vi "MasterAquisitionFile_IOS_Optogenetics_test_no_DigitalOutput.vi"() -> ()   [LabVIEW 2018]
uses:
  <vilib>/vision/driver/IMAQdx.llb/IMAQdx Acquisition Mode.ctl
  <vilib>/vision/driver/IMAQdx.llb/IMAQdx Camera Control Mode.ctl
  <vilib>/userdefined/High Color/IMAQdx.ctl
  <vilib>/vision/driver/IMAQdx.llb/IMAQdx Buffer Number Mode.ctl
  <vilib>/DAQmx/write.llb/DAQmx Write (Analog 2D DBL NChan NSamp).vi
  <vilib>/DAQmx/write.llb/DAQmx Write (Digital Bool 1Line 1Point).vi
  <vilib>/DAQmx/read.llb/DAQmx Read (Analog 1D Wfm NChan NSamp).vi
  <vilib>/DAQmx/create/channels.llb/DAQmx Create Channel (DO-Digital Output).vi
  <vilib>/DAQmx/create/channels.llb/DAQmx Create Channel (AO-Voltage-Basic).vi
  <vilib>/DAQmx/create/channels.llb/DAQmx Create Channel (CO-Pulse Generation-Frequency).vi
  <vilib>/DAQmx/configure/timing.llb/DAQmx Timing (Implicit).vi
  <vilib>/DAQmx/create/channels.llb/DAQmx Create Channel (AI-Voltage-Basic).vi
  <vilib>/DAQmx/configure/timing.llb/DAQmx Timing (Sample Clock).vi
  <vilib>/DAQmx/configure/trigger.llb/DAQmx Start Trigger (Digital Edge).vi
  <vilib>/DAQmx/miscellaneous.llb/DAQmx Fill In Error Info.vi
  <vilib>/vision/driver/NI_Vision_Acquisition_Software.lvlib
  <resource>/objmgr/imaqdx.rc
  <resource>/objmgr/daqmx.rc
panel:
  in  "Solenoid\nPulse Train":bool=TRUE
  out "LED":bool
  out "Auditory":bool
  out "RPad":bool
  out "LPad":bool
  out "Finished":bool
  in  "LED":bool=TRUE
  in  "Sol Stim Parameters":cluster{"Fs":dbl, "Samples":dbl}
  in  "LED Stim Parameters":cluster{"Fs":dbl, "Samples":dbl}
  in  "Sol Duty Cycle (%)":dbl=10.0
  in  "Sol Freq":dbl=1.0
  in  "Sol Dur (s)":dbl=1.0
  in  "LED Duty Cycle (%)":dbl=10.0
  in  "LED Freq":dbl=10.0
  in  "LED Dur (s)":dbl=2.0
  out "Stimulus Order":digitalwaveform[](graph)=[{"t0"=timestamp(0 s since 1904-01-01), "dt"=5e-05, "Y"={"transitions"=[], "data"=array18000000x1[18000000 elements]}}, {"t0"=timestamp(0 s since 1904-01-01), "dt"=5e-05, "Y"={"transitions"=[], "data"=array18000000x1[18000000 elements]}}, {"t0"=timestamp(0 s since 1904-01-01), "dt"=5e-05, "Y"={"transitions"=[], "data"=array18000000x1[18000000 elements]}}, {"t0"=timestamp(0 s since 1904-01-01), "dt"=5e-05, "Y"={"transitions"=[], "data"=array18000000x1[18000000 elements]}}]
  out "Solenoid Stim":digitalwaveform(graph)={"t0"=timestamp(0 s since 1904-01-01), "dt"=5e-05, "Y"={"transitions"=[], "data"=array20000x1[20000 elements]}}
  in  "Trial Offset (s)":dbl=15.0
  in  "Interstim (s)":dbl=30.0
  in  "Right Pad":dbl=1.0
  in  "Left Pad":dbl=1.0
  in  "Auditory":dbl=1.0
  in  "LED":dbl
  out "Dev2 Samples":i32=526603
  out "Dev2 Analog":bool=TRUE
  in  "Dev2 Analog Channels":string[](array[string])=["LD_BackScatter", "LD_Flow", "Opto_LED", "RPadSol", "AudSol", "Hippocampus", "EMG", "Cortical_RH"]
  out "?":T1(plugin-control)
  out "?":T1(plugin-control)
  out "?":T1(plugin-control)
  out "?":T1(plugin-control)
  in  "stop":bool
  out "CBV Cam":bool=TRUE
  out "Pupil Cam":bool=TRUE
  out "Whisk Cam":bool=TRUE
  out "Web Cam":bool=TRUE
  out "Dev1 Analog":bool=TRUE
  out "Web Cam Fs":dbl(knob)=29.14753443801158 scale=0.0..200.0
  out "CBV Cam":dbl(knob)=30.019685039370078 scale=0.0..200.0
  out "Whisk Cam Fs":dbl(knob)=150.04985044865404 scale=0.0..200.0
  out "Last Whisk\nBuffer 2":u32=789
  out "Pupil Cam Fs":dbl(knob)=29.985007496251875 scale=0.0..200.0
  out "Dropped 2":u32(slide) caption="Pupil Cam" scale=0.0..99.0
  in  "Exposure Time (microsec)":string="10000"
  out "Dev1 Samples":i32=526592
  in  "Dev1 Analog Channels":string[](array[string])=["Cortical_LH", "Force_Sensor", "LPadSol", "RPadSol", "AudSol", "Hippocampus", "EMG", "Cortical_RH"]
  in  "Analog Acquisition":cluster{"Analog Fs":u16}={"Analog Fs"=20000} {"Analog Fs" format="%0.0f"}
  in  "Sampling Rates":T2={"CBV Cam Fs"=30, "Whisk Cam Fs"=150, "Web Cam Fs"=15, "Pupil Cam Fs"=30}
  out "Notes Size":i32=8
  out "Notes Reversed":string[](array[string])=["Experimenter", "Animal ID", "Hemisphere", "Solenoid PSI", "Isoflurane time", "Session ID", "Amplifier Gain", "LED power (mW)"]
  out "Notes Array":string[](array[string])=["LED power (mW)", "Amplifier Gain", "Session ID", "Isoflurane time", "Solenoid PSI", "Hemisphere", "Animal ID", "Experimenter"]
  in  "Notes:":T3={"Experimenter"="Kevin", "Animal ID"="T182", "Hemisphere"="Both", "Solenoid PSI"="10", "Isoflurane time"="1030", "Session ID"="Imaging Session Two", "Amplifier Gain"="10000", "LED power (mW)"="0"}
  in  "Target Path":path=path "D:/T182/Imaging Session 2 - 20 Apr. 2021" caption="Final Save Location"
  out "Dropped":u32(slide) caption="Whisk Cam" scale=0.0..999.0
  out "Filename":string="210420_10_44_31"
  out "CBV Camera":bool
  out "Time Elapsed (Min)":cluster{dbl, dbl}(slide)={15.0, 0.43888776} scale=0.0..15.0 scale format="%#_2g"
  in  "Time (min)":dbl(knob)=15.0 min=0.5 max=20.0 step=0.5 scale=0.0..20.0 scale format="%#_2g"
  in  "Temp Path":path=path "D:/LabVIEW Streamed Data" caption="Temporary Path for Streamed Data"
  out "Last CBV\nBuffer":i32=789
  out "Last Whisk\nBuffer":u32=3948
  # "Stimuli"
  # "LPAD"
  # "RPAD"
  # "AUD"
  # "LED"
  # "Ratio"
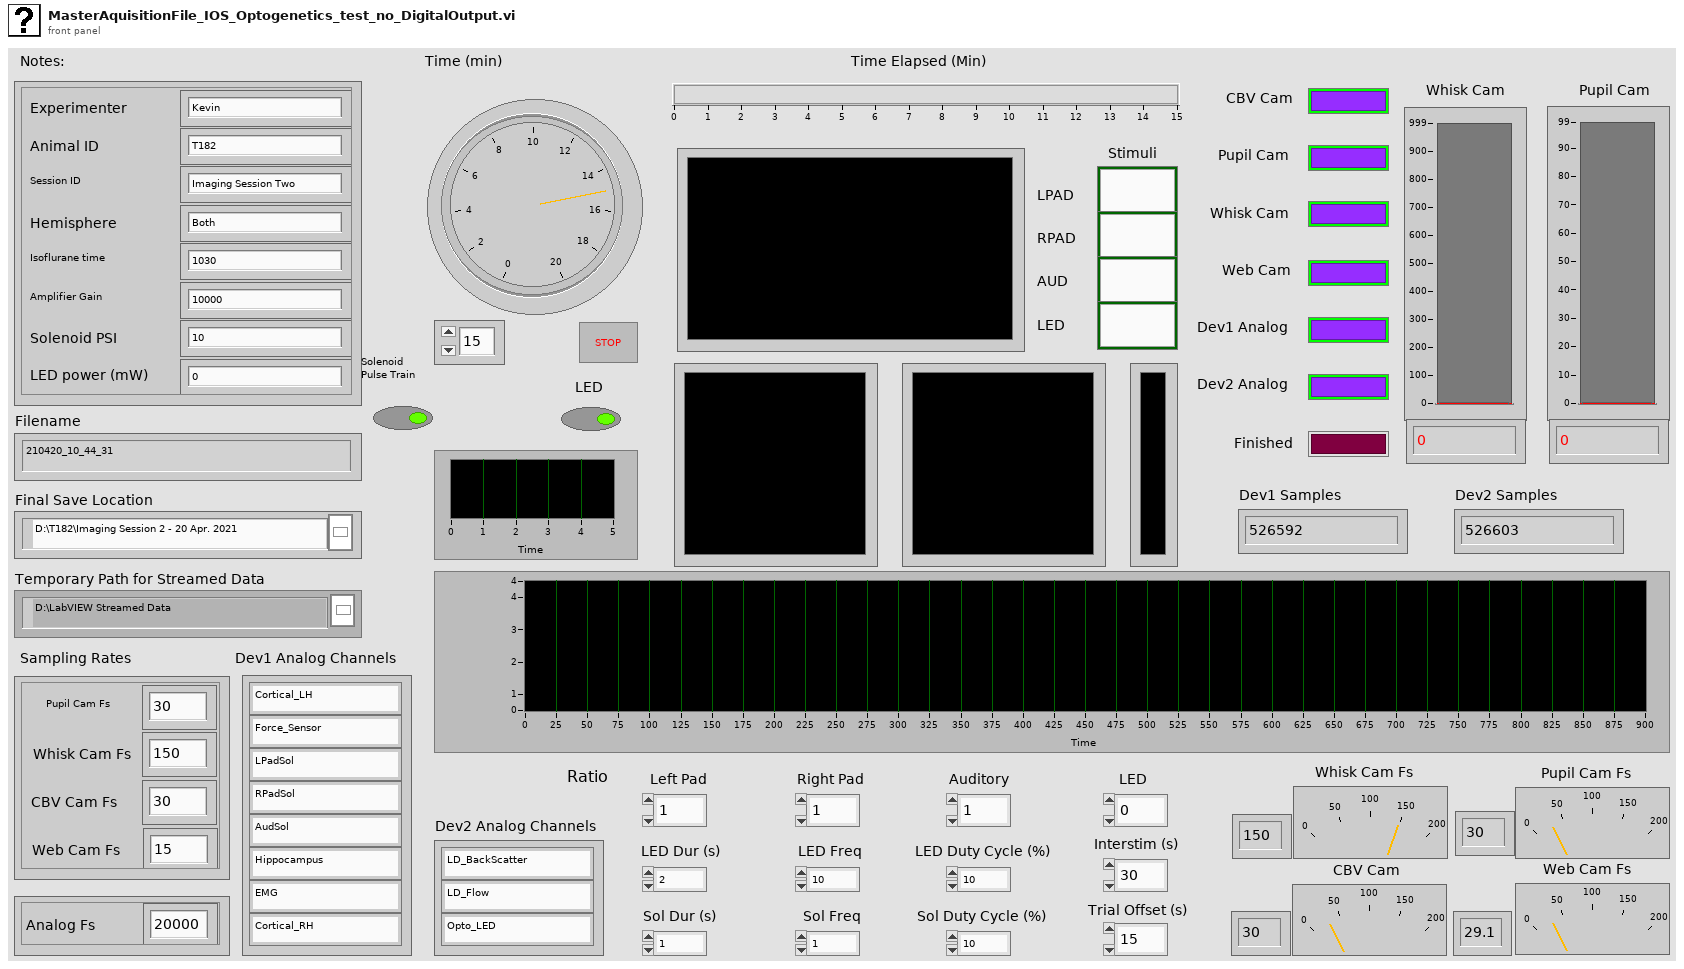
[diagram p1: front panel]
types:
  T1 = typedef "IMAQ Image.ctl" = refnum<image>
  T2 = cluster{"CBV Cam Fs":u16, "Whisk Cam Fs":u16, "Web Cam Fs":u16, "Pupil Cam Fs":u16}
  T3 = cluster{"Experimenter":string, "Animal ID":string, "Hemisphere":string, "Solenoid PSI":string, "Isoflurane time":string, "Session ID":string, "Amplifier Gain":string, "LED power (mW)":string}
  T4 = typedef "IMAQdx.ctl" = refnum<k21>
  T5 = enum16{"open", "open or create", "create or replace", "create", "open (read-only)"}
  T6 = enum16{"open", "replace", "create", "open or create", "replace or create", "replace or create with confirmation"}
  T7 = typedef "Image Type" = u32
  T8 = typedef "NI_Vision_Acquisition_Software.lvlib/IMAQdx Acquisition Mode.ctl" = enum32{"One Shot", "Continuous"}
  T9 = typedef "NI_Vision_Acquisition_Software.lvlib/IMAQdx Camera Control Mode.ctl" = enum32{"Controller", "Listener"}
  T10 = typedef "IMAQ AVI2 Refnum.ctl" = refnum<k20>
  T11 = enum16{"big-endian, network order", "native, host order", "little-endian"}
  T12 = typedef "NI_Vision_Acquisition_Software.lvlib/IMAQdx Buffer Number Mode.ctl" = enum32{"Next", "Last", "Buffer Number", "Every", "Last New"}
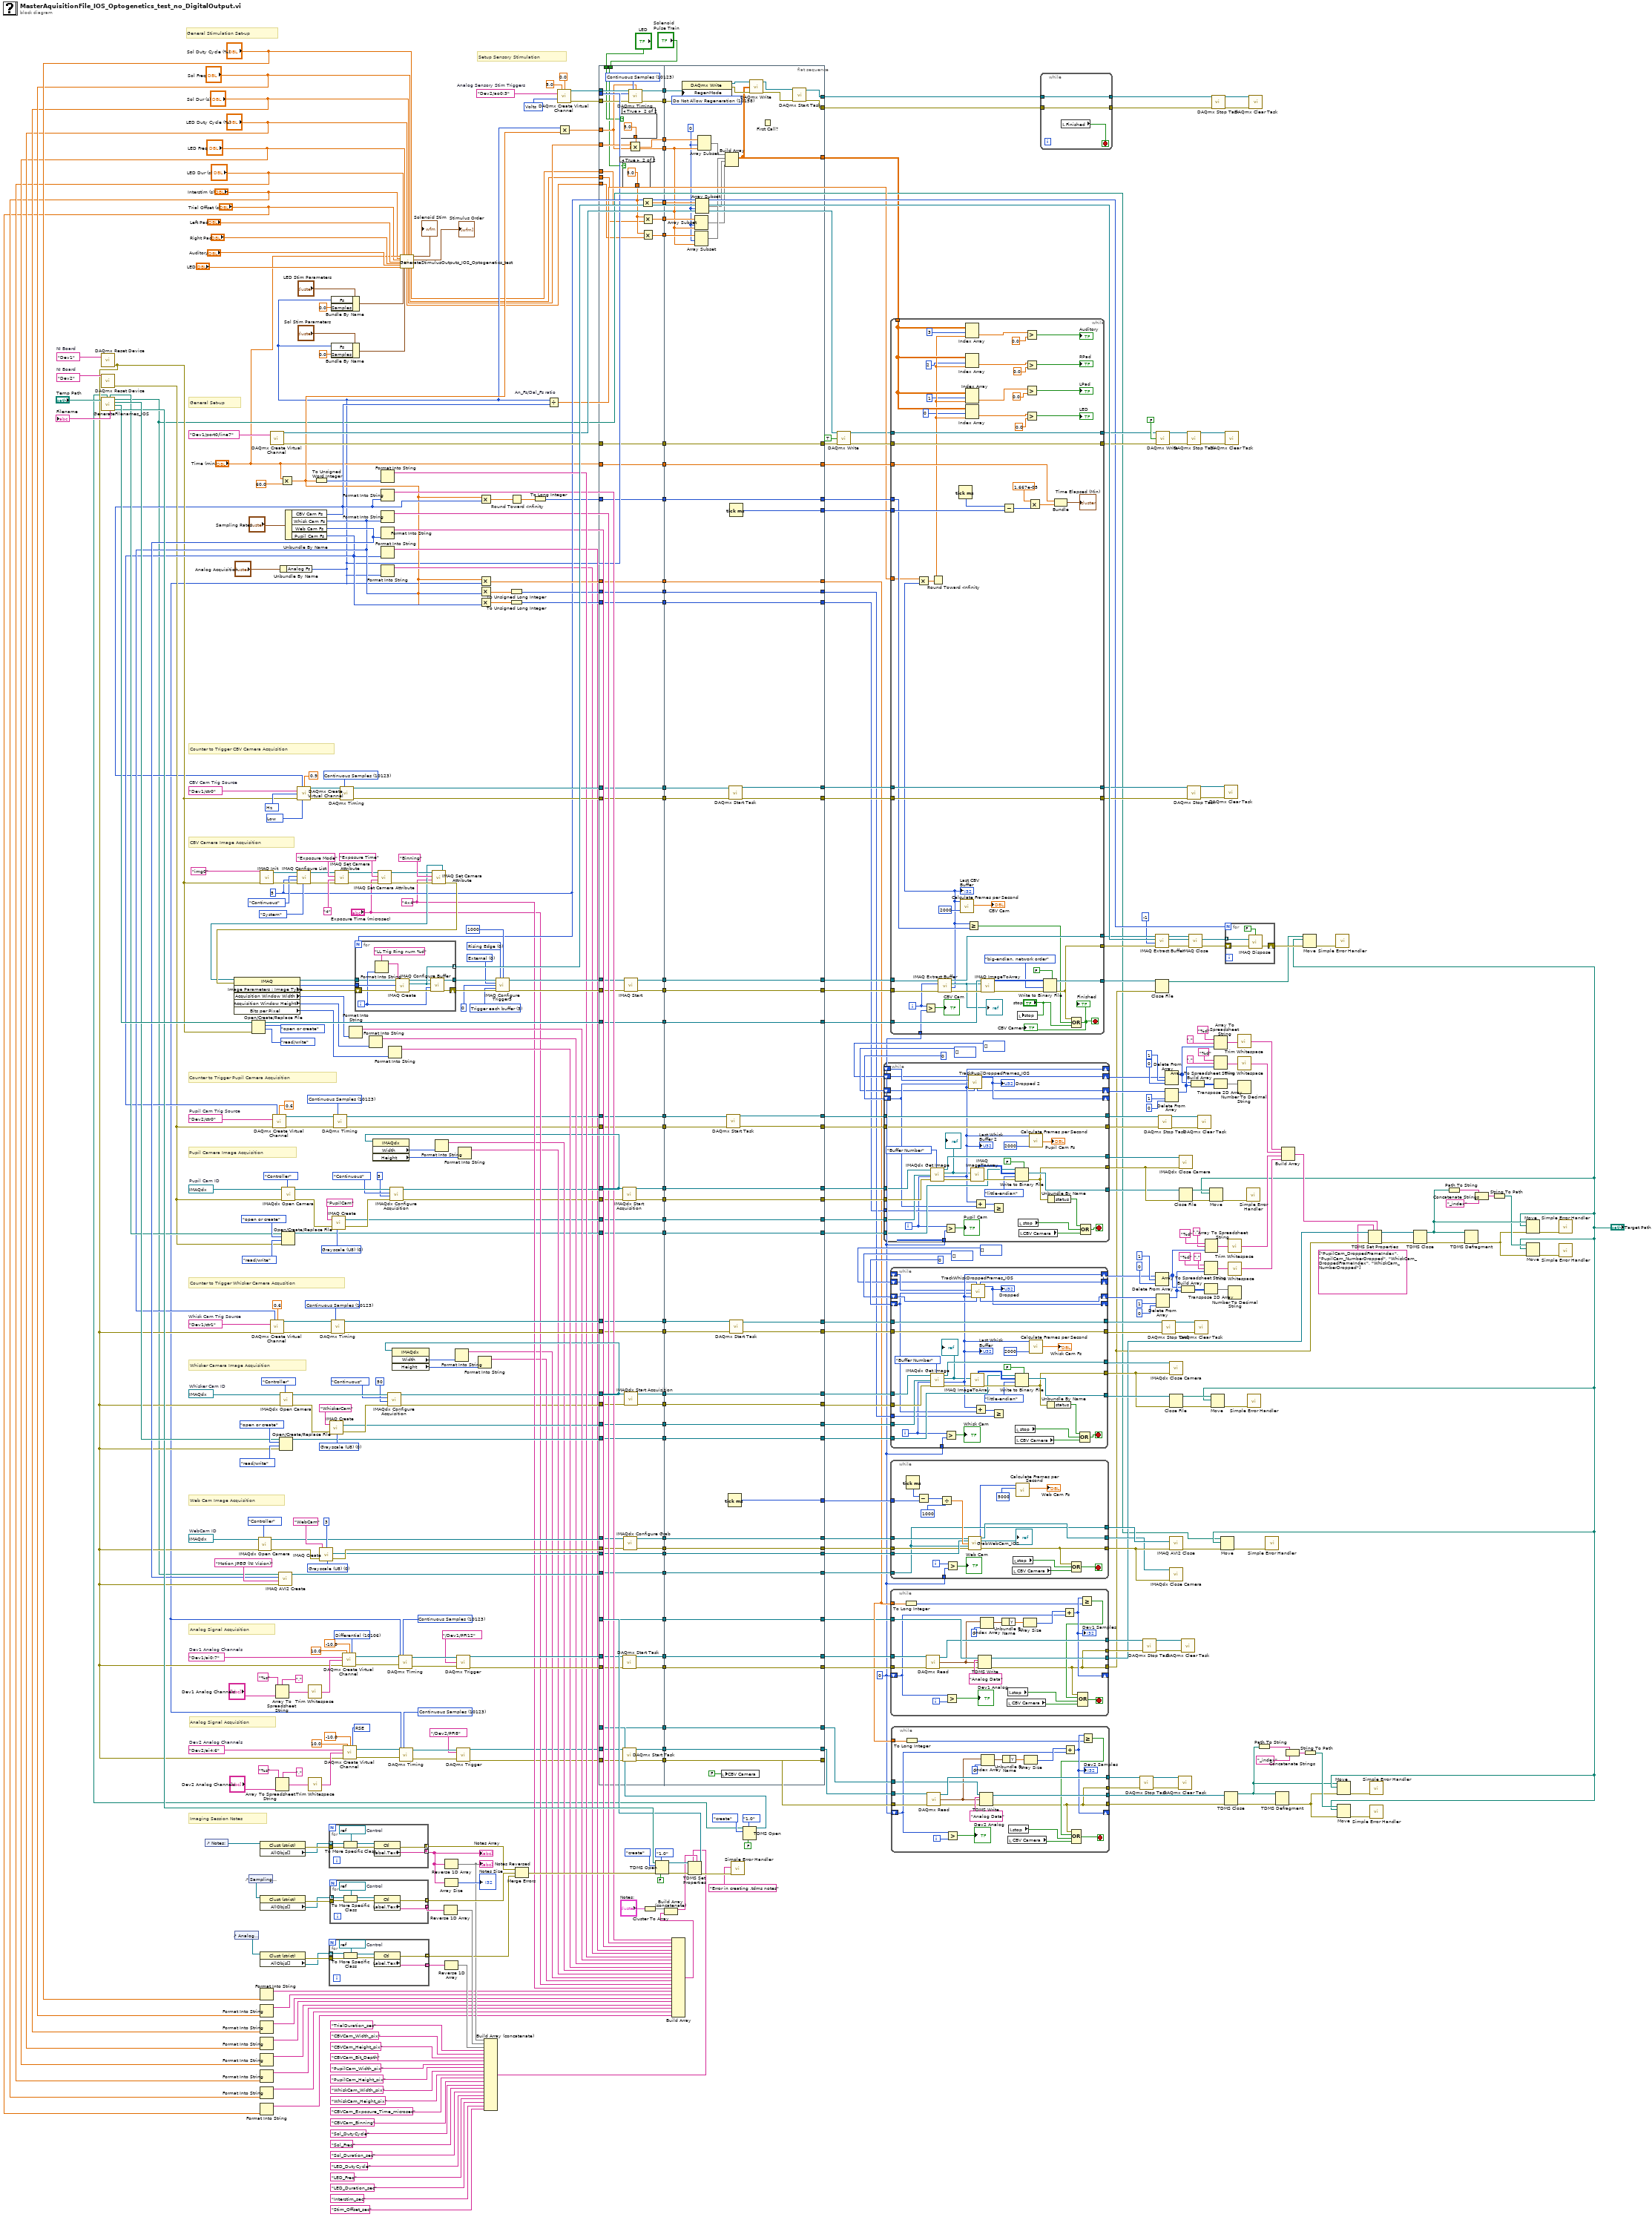
[diagram p0: block diagram]
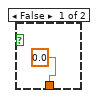
[diagram p2: hidden frame]
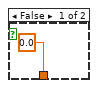
[diagram p3: hidden frame]
diagram:
  w112 = tag "Dev2/ai4:6"  # Dev2 Analog Channels
  w309 = tag "Dev1/ai0:7"  # Dev1 Analog Channels
  w312 = T4 "cam0"  # WebCam ID
  w290 = T4 "cam1"  # Whisker Cam ID
  w484 = tag "Dev1/ctr1"  # Whisk Cam Trig Source
  w212 = T4 "cam2"  # Pupil Cam ID
  w217 = tag "Dev2/ctr0"  # Pupil Cam Trig Source
  w458 = tag "Dev1/ctr0"  # CBV Cam Trig Source
  w58 = 10348 items=["Volts"=10348, "From Custom Scale"=10065] ("units")
  w59 = tag "Dev2/ao0:3"  # Analog Sensory Stim Triggers
  w116 = 10123 items=["Finite Samples"=10178, "Continuous Samples"=10123, "Hardware Timed Single Point"=12522] ("sample mode")
  w119 = 10083 items=["default"=-1, "RSE"=10083, "NRSE"=10078, "Differential"=10106, "Pseudodifferential"=12529] ("input terminal configuration")
  w135 = tag "Dev2"  # NI Board
  w213 = 10123 items=["Finite Samples"=10178, "Continuous Samples"=10123, "Hardware Timed Single Point"=12522] ("sample mode")
  w220 = T7 0 items=["Grayscale (U8)", "Grayscale (I16)", "Grayscale (SGL)", "Complex (CSG)", "RGB (U32)", "HSL (U32)", "RGB (U64)", "Grayscale (U16)"] ("Image Type")
  w202 = "4x4" ("Attribute Value")
  w71 = 0
  w391 = 10123 items=["Finite Samples"=10178, "Continuous Samples"=10123, "Hardware Timed Single Point"=12522] ("sample mode")
  w394 = 10106 items=["default"=-1, "RSE"=10083, "NRSE"=10078, "Differential"=10106, "Pseudodifferential"=12529] ("input terminal configuration")
  w445 = T7 0 items=["Grayscale (U8)", "Grayscale (I16)", "Grayscale (SGL)", "Complex (CSG)", "RGB (U32)", "HSL (U32)", "RGB (U64)", "Grayscale (U16)"] ("Image Type")
  w465 = u32 0 items=["Rising Edge", "Falling Edge"] ("Trigger Polarity")
  w468 = u32 0 items=["External"=0, "RTSI"=1, "ISO In"=2, "Scaled Encoder"=5] ("Trigger Type")
  w459 = tag "Dev1"  # NI Board
  w460 = 10123 items=["Finite Samples"=10178, "Continuous Samples"=10123, "Hardware Timed Single Point"=12522] ("sample mode")
  w463 = 10373 items=["Hz"=10373] ("units")
  w464 = 10214 items=["High"=10192, "Low"=10214] ("idle state")
  w231 = u32 5 ("Number of Buffers")
  w466 = u32 3 items=["Disabled", "Trigger start of acquisition", "Trigger start of each buffer list", "Trigger each buffer", "Trigger each line (linescan)", "Trigger end of acquisition"] ("Action")
  w480 = 10123 items=["Finite Samples"=10178, "Continuous Samples"=10123, "Hardware Timed Single Point"=12522] ("sample mode")
  w487 = T7 0 items=["Grayscale (U8)", "Grayscale (I16)", "Grayscale (SGL)", "Complex (CSG)", "RGB (U32)", "HSL (U32)", "RGB (U64)", "Grayscale (U16)"] ("Image Type")
  # "Setup Sensory Stimulation"
  # "General Stimulation Set-up"
  # "Analog Signal Acquisition"
  # "General Set-up"
  # "Pupil Camera Image Acquisition"
  # "Counter to Trigger Pupil Camera Acquisition"
  # "Whisker Camera Image Acquisition"
  # "Imaging Session Notes"
  # "CBV Camera Image Acquisition"
  # "Counter to Trigger CBV Camera Acquisition"
  # "Counter to Trigger Whisker Camera Acqusition"
  # "Web Cam Image Acquisition"
  # "Analog Signal Acquisition"
  n1 = call <vilib>:"DAQmx Reset Device.vi"("device in"=w459) -> ("error out"=w105:errorcluster)  [unwired: 14 in]
  n2 = call <vilib>:"DAQmx Reset Device.vi"("device in"=w135) -> ("error out"=w134:errorcluster)  [unwired: 14 in]
  n3 = call "GenerateFilenames_IOS.vi"("path"="Temp Path") -> ("TDMS Path"=w334:path, "Dalsa Path"=w452:path, "Basler Path"=w448:path, "WebCam Path"=w41:path, "Analog file name"=→"Filename":string, "Basler2 Path"=w211:path, "TDMS Path 2"=w73:path)  [unwired: 3 in, 1 out]
  n4 = control-ref of="Notes:"() -> (w339:refnum<vi>)
  n5 = control-ref of="Analog Acquisition"() -> (w317:refnum<vi>)
  n6 = control-ref of="Sampling Rates"() -> (w318:refnum<vi>)
  n7 = Open/Create/Replace File(file path (use dialog)=w452, error in=w105, operation (0:open)=T6."open or create", access (0:read/write)=enum16{"read/write", "read-only", "write-only"}."read/write") -> (refnum out=w395:refnum<file>)  [unwired: 2 in, 2 out]
  n8 = call <vilib>:"IMAQdx Open Camera.vi"("Camera Control Mode"=IMAQdx_Camera_Control_Mode."Controller", "error in"=w105, "Session In"=w312) -> ("error out"=w441:errorcluster, "Session Out"=w439:T4)  [unwired: 7 in]
  n9 = property class="Clust (strict)"(reference=w339) -> (error out=w342:errorcluster, "AllObjs[]"=w238:refnum<vi>[])  [unwired: 1 in, 1 out]
  n10 = property class="Clust (strict)"(reference=w318) -> (error out=w337:errorcluster, "AllObjs[]"=w239:refnum<vi>[])  [unwired: 1 in, 1 out]
  n11 = property class="Clust (strict)"(reference=w317) -> (error out=w316:errorcluster, "AllObjs[]"=w237:refnum<vi>[])  [unwired: 1 in, 1 out]
  n12 = call <vilib>:"IMAQ Init.vi"("error in (no error)"=w105, "Interface Name"="img0") -> ("error out"=w478:errorcluster, "IMAQ Session Out"=w479:refnum<k11>)  [unwired: 8 out]
  n13 = Format Into String("Sol Duty Cycle (%)") -> (resulting string=w31:string)  [unwired: 3 in, 1 out]
  n14 = Format Into String("Sol Freq") -> (resulting string=w30:string)  [unwired: 3 in, 1 out]
  n15 = Format Into String("Sol Dur (s)") -> (resulting string=w29:string)  [unwired: 3 in, 1 out]
  n16 = Format Into String("LED Duty Cycle (%)") -> (resulting string=w28:string)  [unwired: 3 in, 1 out]
  n17 = Format Into String("LED Freq") -> (resulting string=w27:string)  [unwired: 3 in, 1 out]
  n18 = Format Into String("LED Dur (s)") -> (resulting string=w26:string)  [unwired: 3 in, 1 out]
  n19 = Format Into String("Interstim (s)") -> (resulting string=w25:string)  [unwired: 3 in, 1 out]
  n20 = Format Into String("Trial Offset (s)") -> (resulting string=w24:string)  [unwired: 3 in, 1 out]
  n21 = call-poly <vilib>:"DAQmx Create Virtual Channel.vi"("lines"=tag "Dev1/port0/line7") -> ("task out"=w268:refnum<k21>, "error out"=w271:errorcluster)  [unwired: 13 in]
  n22 = Array To Spreadsheet String(delimiter (Tab)=",", array="Dev1 Analog Channels", 3:"%s" ("format string")) -> (spreadsheet string=w306:string)
  n23 = Array To Spreadsheet String(delimiter (Tab)=",", array="Dev2 Analog Channels", 3:"%s" ("format string")) -> (spreadsheet string=w109:string)
  n24 = Open/Create/Replace File(file path (use dialog)=w448, error in=w105, operation (0:open)=T6."open or create", access (0:read/write)=enum16{"read/write", "read-only", "write-only"}."read/write") -> (refnum out=w413:refnum<file>)  [unwired: 2 in, 2 out]
  n25 = Unbundle By Name("Analog Acquisition") -> ("Analog Fs"=w15:u16)
  n26 = call <vilib>:"IMAQdx Open Camera.vi"("Camera Control Mode"=IMAQdx_Camera_Control_Mode."Controller", "error in"=w105, "Session In"=w290) -> ("error out"=w490:errorcluster, "Session Out"=w493:T4)  [unwired: 7 in]
  n27 = Multiply(x="Time (min)", y=60.0) -> (x*y=w42:dbl)
  n28 = Open/Create/Replace File(file path (use dialog)=w211, error in=w134, operation (0:open)=T6."open or create", access (0:read/write)=enum16{"read/write", "read-only", "write-only"}."read/write") -> (refnum out=w192:refnum<file>)  [unwired: 2 in, 2 out]
  n29 = call <vilib>:"IMAQdx Open Camera.vi"("Camera Control Mode"=IMAQdx_Camera_Control_Mode."Controller", "error in"=w134, "Session In"=w212) -> ("error out"=w223:errorcluster, "Session Out"=w226:T4)  [unwired: 7 in]
  n30 = Unbundle By Name("Sampling Rates") -> ("CBV Cam Fs"=w46:u16, "Whisk Cam Fs"=w174:u16, "Web Cam Fs"=w311:u16, "Pupil Cam Fs"=w168:u16)
  n31 = call-poly <vilib>:"DAQmx Create Virtual Channel.vi"("frequency"=w174, "duty cycle"=0.6, "counter"=w484, "error in"=w105) -> ("task out"=w482:refnum<k21>, "error out"=w481:errorcluster)  [unwired: 10 in]
  n32 = call-poly <vilib>:"DAQmx Create Virtual Channel.vi"("frequency"=w168, "duty cycle"=0.6, "counter"=w217, "error in"=w134) -> ("task out"=w215:refnum<k21>, "error out"=w214:errorcluster)  [unwired: 10 in]
  n33 = call "IMAQ AVI2 Create"("error in (no error)"=w105, "Codec"="Motion JPEG (NI Vision)", "Frames Per Second"=w311, "AVI Path"=w41) -> ("AVI Refnum"=w431:T10)  [unwired: 6 in, 1 out]
  n34 = call-poly <vilib>:"DAQmx Create Virtual Channel.vi"("frequency"=w46, "duty cycle"=0.9, "counter"=w458, "units"=w463, "error in"=w105, "idle state"=w464) -> ("task out"=w462:refnum<k21>, "error out"=w461:errorcluster)  [unwired: 8 in]
  n35 = call <vilib>:"IMAQ Configure List.vi"("Memory Location"=enum16{"System", "Onboard"}."System", "error in (no error)"=w478, "Number of buffers"=w231, "Continuous?"=enum16{"One-Shot", "Continuous"}."Continuous" ("Continuous ?"), "IMAQ Session In"=w479) -> ("error out"=w252:errorcluster, "IMAQ Session Out"=w248:refnum<k11>)  [unwired: 1 in, 4 out]
  n36 = call <vilib>:"Trim Whitespace.vi"("string"=w306) -> ("trimmed string"=w305:string)  [unwired: 1 in]
  n37 = call <vilib>:"Trim Whitespace.vi"("string"=w109) -> ("trimmed string"=w108:string)  [unwired: 1 in]
  n38 = To Unsigned Word Integer(number=w42) -> (unsigned 16bit integer=w301:u16)
  n39 = call "IMAQ Create"("Border Size"=3, "Image Name"="WebCam", "Image Type"=w445, "error in (no error)"=w441) -> ("New Image"=w438:T1, "error out"=w440:errorcluster)  [unwired: 1 in]
  n40 = for {
    tunnel: [w499] -> w341 mode=indexing
    tunnel: w342 -> [w498]
    tunnel: [w496] -> w325 mode=indexing
    tunnel: w238 -> [w495] mode=indexing
    w500 = refnum<vi> refnum  # Control
    n41 = To More Specific Class(target class=w500, reference=w495, error in=w498) -> (specific class reference=w501:refnum<vi>, error out=w497:errorcluster)
    n42 = property class="Ctl"(reference=w501, error in=w497) -> (error out=w496:errorcluster, "Label.Text"=w499:string)  [unwired: 1 out]
  }
  "Notes Array" <- w341
  n43 = for {
    tunnel: [w506] -> w314 mode=indexing
    tunnel: w316 -> [w505]
    tunnel: [w503] -> w315 mode=indexing
    tunnel: w237 -> [w502] mode=indexing
    w507 = refnum<vi> refnum  # Control
    n44 = To More Specific Class(target class=w507, reference=w502, error in=w505) -> (specific class reference=w508:refnum<vi>, error out=w504:errorcluster)
    n45 = property class="Ctl"(reference=w508, error in=w504) -> (error out=w503:errorcluster, "Label.Text"=w506:string)  [unwired: 1 out]
  }
  n46 = call "IMAQ Create"("Image Name"="WhiskerCam", "Image Type"=w487, "error in (no error)"=w490) -> ("New Image"=w288:T1, "error out"=w488:errorcluster)  [unwired: 2 in]
  n47 = for {
    tunnel: [w513] -> w338 mode=indexing
    tunnel: w337 -> [w512]
    tunnel: [w510] -> w324 mode=indexing
    tunnel: w239 -> [w509] mode=indexing
    w514 = refnum<vi> refnum  # Control
    n48 = To More Specific Class(target class=w514, reference=w509, error in=w512) -> (specific class reference=w515:refnum<vi>, error out=w511:errorcluster)
    n49 = property class="Ctl"(reference=w515, error in=w511) -> (error out=w510:errorcluster, "Label.Text"=w513:string)  [unwired: 1 out]
  }
  n50 = Bundle By Name(cluster="LED Stim Parameters", "Fs"=w15, "Samples"=0.0) -> (w64:cluster{"Fs":dbl, "Samples":dbl})
  n51 = Bundle By Name(cluster="Sol Stim Parameters", "Fs"=w15, "Samples"=0.0) -> (w65:cluster{"Fs":dbl, "Samples":dbl})
  n52 = call-poly <vilib>:"DAQmx Timing.vi"("task/channels in"=w482, "sample mode"=w480, "error in"=w481) -> ("task out"=w376:refnum<k21>, "error out"=w374:errorcluster)  [unwired: 11 in]
  n53 = call "IMAQ Create"("Image Name"="PupilCam", "Image Type"=w220, "error in (no error)"=w223) -> ("New Image"=w177:T1, "error out"=w221:errorcluster)  [unwired: 2 in]
  n54 = call-poly <vilib>:"DAQmx Timing.vi"("task/channels in"=w215, "sample mode"=w213, "error in"=w214) -> ("task out"=w190:refnum<k21>, "error out"=w188:errorcluster)  [unwired: 11 in]
  n55 = call <vilib>:"IMAQ Set Camera Attribute.vi"("error in (no error)"=w252, "Attribute Value"="4", "Camera Attribute"="Exposure Mode", "IMAQ Session In"=w248) -> ("error out"=w251:errorcluster, "IMAQ Session Out"=w247:refnum<k11>)  [unwired: 4 in]
  n56 = call-poly <vilib>:"DAQmx Timing.vi"("task/channels in"=w462, "sample mode"=w460, "error in"=w461) -> ("task out"=w380:refnum<k21>, "error out"=w378:errorcluster)  [unwired: 11 in]
  n57 = call-poly <vilib>:"DAQmx Create Virtual Channel.vi"("maximum value"=10.0, "minimum value"=-10.0, "input terminal configuration"=w394, "physical channels"=w309, "name to assign"=w305, "error in"=w105) -> ("task out"=w393:refnum<k21>, "error out"=w392:errorcluster)  [unwired: 8 in]
  n58 = call-poly <vilib>:"DAQmx Create Virtual Channel.vi"("maximum value"=10.0, "minimum value"=-10.0, "input terminal configuration"=w119, "physical channels"=w112, "name to assign"=w108, "error in"=w105) -> ("task out"=w118:refnum<k21>, "error out"=w117:errorcluster)  [unwired: 8 in]
  n59 = call <vilib>:"IMAQ Set Camera Attribute.vi"("error in (no error)"=w251, "Attribute Value"="Exposure Time (microsec)", "Camera Attribute"="Exposure Time", "IMAQ Session In"=w247) -> ("error out"=w250:errorcluster, "IMAQ Session Out"=w246:refnum<k11>)  [unwired: 4 in]
  n60 = Format Into String(w301) -> (resulting string=w303:string)  [unwired: 3 in, 1 out]
  n61 = Format Into String(w46) -> (resulting string=w172:string)  [unwired: 3 in, 1 out]
  n62 = Format Into String(w174) -> (resulting string=w171:string)  [unwired: 3 in, 1 out]
  n63 = Format Into String(w311) -> (resulting string=w170:string)  [unwired: 3 in, 1 out]
  n64 = Format Into String(w168) -> (resulting string=w121:string)  [unwired: 3 in, 1 out]
  n65 = Format Into String(w15) -> (resulting string=w120:string)  [unwired: 3 in, 1 out]
  n66 = call <vilib>:"IMAQdx Configure Acquisition.vi"("error in"=w488, "Number of Buffers"=u32 50, "Continuous?"=IMAQdx_Acquisition_Mode."Continuous", "Session In"=w493) -> ("error out"=w136:errorcluster, "Session Out"=w289:T4)  [unwired: 6 in]
  n67 = call <vilib>:"IMAQdx Configure Acquisition.vi"("error in"=w221, "Number of Buffers"=u32 5, "Continuous?"=IMAQdx_Acquisition_Mode."Continuous", "Session In"=w226) -> ("error out"=w194:errorcluster, "Session Out"=w178:T4)  [unwired: 6 in]
  n68 = property class="IMAQdx"(reference=w178) -> ("Width"=w210:u32, "Height"=w209:u32)  [unwired: 1 in, 2 out]
  n69 = property class="IMAQdx"(reference=w289) -> ("Width"=w300:u32, "Height"=w299:u32)  [unwired: 1 in, 2 out]
  n70 = call-poly <vilib>:"DAQmx Timing.vi"("task/channels in"=w393, "sample mode"=w391, "rate"=w15, "error in"=w392) -> ("task out"=w235:refnum<k21>, "error out"=w390:errorcluster)  [unwired: 10 in]
  n71 = call-poly <vilib>:"DAQmx Timing.vi"("task/channels in"=w118, "sample mode"=w116, "rate"=w15, "error in"=w117) -> ("task out"=w106:refnum<k21>, "error out"=w115:errorcluster)  [unwired: 10 in]
  n72 = call "GenerateStimulusOutputs_IOS_Optogenetics_test.vi"("Trial duration (min)"="Time (min)", "Rest duration(s)"="Interstim (s)", "trial offset (s)"="Trial Offset (s)", "Left Pad"="Left Pad", "Right Pad"="Right Pad", "Auditory"="Auditory", "LED"="LED", "LED Stim Duration (s)"="LED Dur (s)", "LED Stim Parameters"=w64, "LED Frequency"="LED Freq", "Sol Stim Parameters"=w65, "LED duty cycle (%)"="LED Duty Cycle (%)", "Sol Stim Duration (s)"="Sol Dur (s)", "Sol Frequency"="Sol Freq", "Sol Duty Cycle (%)"="Sol Duty Cycle (%)") -> ("Double Left Puff"=w10:dbl[], "Double LED Out"=w12:dbl[], "Double Control Puff"=w9:dbl[], "Double Right Puff"=w8:dbl[], "Solenoid Stim Waveforms"=→"Solenoid Stim":digitalwaveform, "Stimulus Digital Outputs"=→"Stimulus Order":digitalwaveform[])  [unwired: 3 in, 4 out]
  n73 = call <vilib>:"IMAQ Set Camera Attribute.vi"("error in (no error)"=w250, "Attribute Value"=w202, "Camera Attribute"="Binning", "IMAQ Session In"=w246) -> ("error out"=w249:errorcluster, "IMAQ Session Out"=w245:refnum<k11>)  [unwired: 4 in]
  n74 = property class="IMAQ"(reference=w245, error in=w249) -> (reference out=w259:refnum<k11>, error out=w258:errorcluster, "Image Parameters : Image Type"=w474:u32, "Acquisition Window Width"=w298:u32, "Acquisition Window Height"=w297:u32, "Bits per Pixel"=w296:u32)
  n75 = Format Into String(w298) -> (resulting string=w295:string)  [unwired: 3 in, 1 out]
  n76 = for {
    N: w231 -> [_]
    tunnel: [w525] -> w470
    tunnel: w474 -> [w523]
    shift-right: [w524] -> w469
    shift-left: w258 -> [w522]
    tunnel: [w517] -> w471 mode=indexing
    tunnel: w259 -> [w516]
    i -> [w518]
    n77 = Format Into String(format string="LL Trig Ring num %d", w518) -> (resulting string=w520:string)  [unwired: 2 in, 1 out]
    n78 = call "IMAQ Create"("Image Name"=w520, "Image Type"=w523, "error in (no error)"=w522) -> ("New Image"=w517:T1, "error out"=w521:errorcluster)  [unwired: 1 in, 1 out]
    n79 = call <vilib>:"IMAQ Configure Buffer.vi"("error in (no error)"=w521, "Buffer Number"=w518, "Image In"=w517, "IMAQ Session In"=w516) -> ("error out"=w524:errorcluster, "IMAQ Session Out"=w525:refnum<k11>)  [unwired: 2 in, 4 out]
  }
  n80 = Format Into String(w297) -> (resulting string=w232:string)  [unwired: 3 in, 1 out]
  n81 = Format Into String(w296) -> (resulting string=w294:string)  [unwired: 3 in, 1 out]
  n82 = Format Into String(w210) -> (resulting string=w197:string)  [unwired: 3 in, 1 out]
  n83 = Reverse 1D Array(array=w338) -> (reversed array=w328:string[])
  n84 = Reverse 1D Array(array=w341) -> (reversed array=w236:string[])
  "Notes Reversed" <- w236
  n85 = Array Size(array=w341) -> (size(s)=→"Notes Size":i32)
  n86 = Reverse 1D Array(array=w314) -> (reversed array=w313:string[])
  n87 = Format Into String(w300) -> (resulting string=w199:string)  [unwired: 3 in, 1 out]
  n88 = call-poly <vilib>:"DAQmx Trigger.vi"("task/channels in"=w235, "source"=tag "/Dev1/PFI12", "error in"=w390) -> ("task out"=w389:refnum<k21>, "error out"=w388:errorcluster)  [unwired: 11 in]
  n89 = call-poly <vilib>:"DAQmx Trigger.vi"("task/channels in"=w106, "source"=tag "/Dev2/PFI8", "error in"=w115) -> ("task out"=w104:refnum<k21>, "error out"=w103:errorcluster)  [unwired: 11 in]
  n90 = Format Into String(w209) -> (resulting string=w198:string)  [unwired: 3 in, 1 out]
  n91 = Format Into String(w299) -> (resulting string=w200:string)  [unwired: 3 in, 1 out]
  n92 = Multiply(x=w42, y=w46) -> (x*y=w450:dbl)
  n93 = Multiply(x=w42, y=w15) -> (x*y=w277:dbl)
  n94 = Multiply(x=w174, y=w42) -> (x*y=w233:dbl)
  n95 = Multiply(x=w168, y=w42) -> (x*y=w173:dbl)
  n96 = Build Array (concatenate)(w236, w328, w313, "TrialDuration_sec", "CBVCam_Width_pix", "CBVCam_Height_pix", "CBVCam_Bit_Depth", "PupilCam_Width_pix", "PupilCam_Height_pix", "WhiskCam_Width_pix", "WhiskCam_Height_pix", "CBVCam_Exposure_Time_microsec" ("element"), "CBVCam_Binning" ("element"), "Sol_DutyCycle", "Sol_Freq", "Sol_Duration_sec", "LED_DutyCycle", "LED_Freq", "LED_Duration_sec", "Interstim_sec", "Stim_Offset_sec") -> (w228:string[])
  n97 = call <vilib>:"IMAQ Configure Trigger3.vi"("IMAQ Session In"=w470, "Polarity"=w465, "Frame timeout (ms)"=u32 1000 ("Frame Timeout (ms)"), "Type"=w468, "Line Number"=u32 0 ("Trigger Line Number"), "Action"=w466, "error in (no error)"=w469) -> ("IMAQ Session Out"=w412:refnum<k11>, "error out"=w411:errorcluster)  [unwired: 2 in, 5 out]
  n98 = To Unsigned Long Integer(number=w233) -> (unsigned 32bit integer=w275:u32)
  n99 = To Unsigned Long Integer(number=w173) -> (unsigned 32bit integer=w169:u32)
  n100 = Round Toward -Infinity(1:w450) -> (0:w449:dbl)
  n101 = Merge Errors(w325, w324, w315) -> (w323:errorcluster)
  n102 = To Long Integer(number=w449) -> (32bit integer=w137:i32)
  n103 = Divide "An_Fs/Dal_Fs ratio"(x=w15, y=w46) -> (x/y=w45:dbl)
  n104 = call-poly <vilib>:"DAQmx Create Virtual Channel.vi"("maximum value"=5.0, "minimum value"=0.0, "physical channels"=w59, "units"=w58) -> ("task out"=w50:refnum<k21>, "error out"=w47:errorcluster)  [unwired: 10 in]
  n105 = Multiply(x=w15, y=w42) -> (x*y=w52:dbl)
  n106 = flat-sequence {
    tunnel: w440 -> [w589]
    tunnel: w439 -> [w588]
    tunnel: w438 -> [w587]
    tunnel: [w587] -> w437
    tunnel: [w586] -> w435
    tunnel: [w585] -> w433
    tunnel: w431 -> [w584]
    tunnel: [w584] -> w430
    tunnel: w289 -> [w583]
    tunnel: w136 -> [w582]
    tunnel: [w581] -> w420
    tunnel: [w580] -> w418
    tunnel: [w579] -> w416
    tunnel: w288 -> [w579]
    tunnel: [w578] -> w414
    tunnel: w413 -> [w578]
    tunnel: w412 -> [w577]
    tunnel: w411 -> [w576]
    tunnel: [w575] -> w409
    tunnel: [w574] -> w407
    tunnel: w137 -> [w573]
    tunnel: [w573] -> w401
    tunnel: "Time (min)" -> [w572]
    tunnel: [w572] -> w398
    tunnel: [w571] -> w396
    tunnel: w395 -> [w571]
    tunnel: w389 -> [w570]
    tunnel: w388 -> [w569]
    tunnel: [w568] -> w387
    tunnel: [w567] -> w386
    tunnel: [w566] -> w382
    tunnel: w326 -> [w566]
    tunnel: w380 -> [w565]
    tunnel: [w565] -> w379
    tunnel: w378 -> [w564]
    tunnel: [w564] -> w377
    tunnel: w376 -> [w563]
    tunnel: [w563] -> w375
    tunnel: w374 -> [w562]
    tunnel: [w562] -> w373
    tunnel: w277 -> [w561]
    tunnel: [w561] -> w276
    tunnel: w275 -> [w560]
    tunnel: [w560] -> w274
    tunnel: w271 -> [w559]
    tunnel: [w559] -> w270
    tunnel: [w552] -> w196
    tunnel: w178 -> [w553]
    tunnel: [w550] -> w195
    tunnel: w194 -> [w551]
    tunnel: [w558] -> w193
    tunnel: w192 -> [w558]
    tunnel: [w557] -> w191
    tunnel: w190 -> [w557]
    tunnel: [w556] -> w189
    tunnel: w188 -> [w556]
    tunnel: w177 -> [w555]
    tunnel: [w555] -> w176
    tunnel: w169 -> [w554]
    tunnel: [w554] -> w167
    tunnel: w104 -> [w549]
    tunnel: w103 -> [w548]
    tunnel: [w547] -> w102
    tunnel: [w546] -> w101
    tunnel: w76 -> [w545]
    tunnel: [w545] -> w75
    tunnel: w12 -> [w543]
    tunnel: [w542] -> w53
    tunnel: w52 -> [w536]
    tunnel: [w536] -> w51
    tunnel: w50 -> [w541]
    tunnel: [w540] -> w49
    tunnel: [w539] -> w48
    tunnel: w47 -> [w538]
    tunnel: w15 -> [w537]
    tunnel: "LED" -> [w535]
    tunnel: "Solenoid\nPulse Train" -> [w533]
    tunnel: w10 -> [w531]
    tunnel: w9 -> [w530]
    tunnel: w8 -> [w529]
    tunnel: [w528] -> w7
    tunnel: [w527] -> w6
    tunnel: [w526] -> w5
    tunnel: [w655] -> w442
    tunnel: w437 -> [w654]
    tunnel: [w654] -> w436
    tunnel: w435 -> [w653]
    tunnel: [w653] -> w434
    tunnel: w433 -> [w652]
    tunnel: [w652] -> w432
    tunnel: w430 -> [w651]
    tunnel: [w651] -> w429
    tunnel: [w633] -> w426
    tunnel: [w632] -> w424
    tunnel: [w650] -> w421
    tunnel: w420 -> [w650]
    tunnel: [w649] -> w419
    tunnel: w418 -> [w649]
    tunnel: [w648] -> w417
    tunnel: w416 -> [w648]
    tunnel: [w647] -> w415
    tunnel: w414 -> [w647]
    tunnel: [w646] -> w410
    tunnel: w409 -> [w646]
    tunnel: [w645] -> w408
    tunnel: w407 -> [w645]
    tunnel: [w637] -> w405
    tunnel: [w636] -> w403
    tunnel: [w644] -> w402
    tunnel: w401 -> [w643]
    tunnel: [w643] -> w400
    tunnel: [w642] -> w399
    tunnel: w398 -> [w642]
    tunnel: [w641] -> w397
    tunnel: w396 -> [w641]
    tunnel: [w640] -> w384
    tunnel: w387 -> [w640]
    tunnel: [w639] -> w385
    tunnel: w386 -> [w639]
    tunnel: [w638] -> w99
    tunnel: w382 -> [w638]
    tunnel: w379 -> [w635]
    tunnel: w377 -> [w634]
    tunnel: w375 -> [w631]
    tunnel: w373 -> [w630]
    tunnel: w276 -> [w629]
    tunnel: [w629] -> w100
    tunnel: w274 -> [w628]
    tunnel: [w628] -> w166
    tunnel: w270 -> [w627]
    tunnel: [w627] -> w269
    tunnel: w196 -> [w625]
    tunnel: w195 -> [w624]
    tunnel: w193 -> [w623]
    tunnel: w191 -> [w620]
    tunnel: w189 -> [w619]
    tunnel: [w617] -> w184
    tunnel: [w618] -> w183
    tunnel: [w625] -> w182
    tunnel: [w624] -> w181
    tunnel: [w623] -> w180
    tunnel: [w622] -> w175
    tunnel: w176 -> [w622]
    tunnel: [w621] -> w165
    tunnel: w167 -> [w621]
    tunnel: [w616] -> w97
    tunnel: w102 -> [w616]
    tunnel: [w615] -> w98
    tunnel: w101 -> [w615]
    tunnel: [w614] -> w74
    tunnel: w75 -> [w614]
    tunnel: w53 -> [w612]
    tunnel: w51 -> [w606]
    tunnel: w49 -> [w611]
    tunnel: w48 -> [w610]
    tunnel: w7 -> [w609]
    tunnel: w6 -> [w608]
    tunnel: w5 -> [w607]
    tunnel: [w598] -> w3
    tunnel: [w595] -> w2
    tunnel: [w594] -> w1
    frame #0 {
      w544 = 10123 items=["Finite Samples"=10178, "Continuous Samples"=10123, "Hardware Timed Single Point"=12522] ("sample mode")
      n107 = case shown="True" w535 {
        tunnel: [0.0 5.0] -> w534
        frame False {
        }
        frame True {
        }
      }
      n108 = call <vilib>:"IMAQdx Start Acquisition.vi"("error in"=w551, "Session In"=w553) -> ("error out"=w550:errorcluster, "Session Out"=w552:T4)  [unwired: 8 in]
      n109 = call <vilib>:"DAQmx Start Task.vi"("task/channels in"=w570, "error in"=w569) -> ("task out"=w568:refnum<k21>, "error out"=w567:errorcluster)  [unwired: 12 in]
      n110 = call <vilib>:"DAQmx Start Task.vi"("task/channels in"=w549, "error in"=w548) -> ("task out"=w546:refnum<k21>, "error out"=w547:errorcluster)  [unwired: 12 in]
      n111 = case shown="True" w533 {
        tunnel: [0.0 5.0] -> w532
        frame False {
        }
        frame True {
        }
      }
      n112 = call <vilib>:"IMAQdx Configure Grab.vi"("error in"=w589, "Session In"=w588) -> ("error out"=w585:errorcluster, "Session Out"=w586:T4)  [unwired: 8 in]
      n113 = call <vilib>:"IMAQ Start.vi"("error in (no error)"=w576, "IMAQ Session In"=w577) -> ("error out"=w574:errorcluster, "IMAQ Session Out"=w575:refnum<k11>)  [unwired: 8 out]
      n114 = call <vilib>:"IMAQdx Start Acquisition.vi"("error in"=w582, "Session In"=w583) -> ("error out"=w580:errorcluster, "Session Out"=w581:T4)  [unwired: 8 in]
      n115 = call-poly <vilib>:"DAQmx Timing.vi"("task/channels in"=w541, "sample mode"=w544, "samples per channel"=w536, "rate"=w537, "error in"=w538) -> ("task out"=w540:refnum<k21>, "error out"=w539:errorcluster)  [unwired: 9 in]
      n116 = Multiply(x=w543, y=w534) -> (x*y=w542:dbl[])
      n117 = Multiply(x=w532, y=w529) -> (x*y=w528:dbl[])
      n118 = Multiply(x=w532, y=w530) -> (x*y=w527:dbl[])
      n119 = Multiply(x=w532, y=w531) -> (x*y=w526:dbl[])
    }
    frame #1 {
      w613 = 10158 items=["Allow Regeneration"=10097, "Do Not Allow Regeneration"=10158] ("RegenMode")
      w605 = 0 ("index")
      n120 = property class="DAQmx Write"(reference=w611, error in=w610, "RegenMode"=w613) -> (reference out=w600:refnum<k21>, error out=w599:errorcluster)
      n121 = Array Subset(array=w608, index=w605, length=w606) -> (w601:dbl[])
      n122 = Array Subset(array=w607, index=w605, length=w606) -> (w603:dbl[])
      n123 = Array Subset(array=w609, index=w605, length=w606) -> (w602:dbl[])
      n124 = Array Subset(array=w612, index=w605, length=w606) -> (w604:dbl[])
      n125 = local write "CBV Camera"(FALSE ("Finished Acquiring")) -> ()
      n126 = Build Array(w604, w603, w602, w601) -> (w598:dbl[][])
      n127 = call <vilib>:"DAQmx Start Task.vi"("task/channels in"=w620, "error in"=w619) -> ("task out"=w617:refnum<k21>, "error out"=w618:errorcluster)  [unwired: 12 in]
      n128 = Tick Count (ms)() -> (millisecond timer value=w655:u32)
      n129 = call <vilib>:"DAQmx Start Task.vi"("task/channels in"=w635, "error in"=w634) -> ("task out"=w637:refnum<k21>, "error out"=w636:errorcluster)  [unwired: 12 in]
      n130 = call <vilib>:"DAQmx Start Task.vi"("task/channels in"=w631, "error in"=w630) -> ("task out"=w633:refnum<k21>, "error out"=w632:errorcluster)  [unwired: 12 in]
      n131 = Tick Count (ms)() -> (millisecond timer value=w644:u32)
      n132 = call-poly <vilib>:"DAQmx Write.vi"("task/channels in"=w600, "data"=w598, "error in"=w599) -> ("task out"=w597:refnum<k21>, "error out"=w596:errorcluster)  [unwired: 10 in, 1 out]
      n133 = First Call?() -> ()  [unwired: 1 out]
      n134 = call <vilib>:"DAQmx Start Task.vi"("task/channels in"=w597, "error in"=w596) -> ("task out"=w595:refnum<k21>, "error out"=w594:errorcluster)  [unwired: 12 in]
    }
  }
  n135 = Cluster To Array(cluster="Notes:") -> (array=w335:string[])
  n136 = TDMS Open(6:FALSE ("disable buffering? (T)"), 7:enum16{"1.0", "2.0"}."1.0" ("file format version (2.0)"), 8:w323, 10:T5."create" ("operation (0:open)"), 11:w334) -> (0:w329:errorcluster, 3:w330:refnum<k34>)  [unwired: 2 in]
  n137 = Build Array(w172, w171, w170, w121, w120, w303, w295, w232, w294, w197, w198, w199, w200, "Exposure Time (microsec)", w202, w31, w30, w29, w28, w27, w26, w25, w24) -> (w310:string[])
  n138 = Build Array (concatenate)(w335, w310) -> (w327:string[])
  n139 = TDMS Set Properties(5:w327, 7:w228, 8:w329, 11:w330) -> (0:w322:errorcluster, 3:w326:refnum<k34>)  [unwired: 2 in, 2 out]
  n140 = call <vilib>:"Simple Error Handler.vi"("error source (\" \")"="Error in creating .tdms notes" ("error source (\" \")"), "error in (no error)"=w322) -> ()  [unwired: 3 in, 5 out]
  n141 = TDMS Open(6:FALSE ("disable buffering? (T)"), 7:enum16{"1.0", "2.0"}."1.0" ("file format version (2.0)"), 10:T5."create" ("operation (0:open)"), 11:w73) -> (3:w76:refnum<k34>)  [unwired: 3 in, 1 out]
  n142 = call-poly <vilib>:"DAQmx Write.vi"("task/channels in"=w268, "data"=TRUE, "error in"=w269) -> ("task out"=w4:refnum<k21>, "error out"=w265:errorcluster)  [unwired: 10 in, 1 out]
  n143 = while {
    tunnel: w184 -> [w681]
    tunnel: [w682] -> w150
    tunnel: w183 -> [w682]
    tunnel: [w681] -> w149
    tunnel: [w670] -> w147
    tunnel: [w671] -> w148
    tunnel: [w680] -> w146
    tunnel: w182 -> [w679]
    tunnel: w181 -> [w678]
    tunnel: w175 -> [w677]
    tunnel: w180 -> [w676]
    shift-right: [w669] -> _
    shift-left: _ -> [w675]
    shift-right: [w674] -> _
    shift-left: u32 0 ("New Lost") -> [w668]
    shift-right: [w673] -> w144
    shift-left: u32[] [] ("NewBuffNum") -> [w664]
    shift-right: [w672] -> w145
    shift-left: u32[] [] ("NewNumLost") -> [w665]
    tunnel: w165 -> [w663]
    tunnel: w71 -> [w661]
    i -> [w656]
    stop <- w666 stop-if-true
    n144 = call <vilib>:"IMAQdx Get Image.vi"("Buffer Number Mode (Next)"=IMAQdx_Buffer_Number_Mode."Buffer Number", "error in"=w678, "Buffer Number In"=w656, "Image In"=w677, "Session In"=w679) -> ("error out"=w689:errorcluster, "Buffer Number Out"=w669:u32, "Image Out"=w658:T1, "Session Out"=w670:T4)  [unwired: 3 in]
    "Last Whisk\nBuffer 2" <- w669
    "?" <- w658
    n145 = Greater?(x=w656, y=w661) -> (0:→"Pupil Cam":bool)
    n146 = call "TrackPupilDroppedFrames_IOS.vi"("NumLost"=w665, "BuffNum"=w664, "Curr Buffer"=w669, "Prev Lost"=w668, "Prev Buffer"=w675) -> ("New Lost"=w674:u32, "NewNumLost"=w672:u32[], "NewBuffNum"=w673:u32[])  [unwired: 4 in]
    "Dropped 2" <- w674
    n147 = call "IMAQ ImageToArray"("error in (no error)"=w689, "Image"=w658) -> ("error out"=w688:errorcluster, "Image Pixels (U8)"=w687:u8[][])  [unwired: 2 in, 3 out]
    n148 = Add(x=w669, y=w668) -> (x+y=w667:u32)
    n149 = Greater Or Equal?(x=w667, y=w663) -> ()  [unwired: 1 out]
    n150 = Write to Binary File(file (use dialog)=w676, data=w687, error in=w688, 5:FALSE ("prepend array or string size? (T)"), 9:T11."little-endian" ("byte order (0:big-endian, network order)")) -> (refnum out=w680:refnum<file>, error out=w671:errorcluster)  [unwired: 1 in, 1 out]
    n151 = local read "stop"() -> (w660:bool)
    n152 = local read "CBV Camera"() -> (w659:bool)
    n153 = call <vilib>:"Calculate Frames per Second.vi"("Update Interval (ms)"=u32 2000, "Buffer Number"=w669) -> ("Processed Frames/s"=→"Pupil Cam Fs":dbl)  [unwired: 7 in, 2 out]
    n154 = Unbundle By Name(w671) -> ("status"=w657:bool)
    n155 = Compound Arithmetic op=OR(w657, w660, w659) -> (w666:bool)
  }
  n156 = while {
    tunnel: w410 -> [w742]
    tunnel: w408 -> [w743]
    tunnel: [w723] -> w454
    tunnel: [w721] -> w455
    tunnel: [w737] -> w453
    tunnel: [w732] -> w406
    tunnel: w405 -> [w732]
    tunnel: [w731] -> w404
    tunnel: w403 -> [w731]
    tunnel: w402 -> [w730]
    tunnel: w400 -> [w729]
    tunnel: w399 -> [w728]
    tunnel: w397 -> [w720]
    tunnel: w4 -> [w725]
    tunnel: [w725] -> w266
    tunnel: [w724] -> w264
    tunnel: w265 -> [w724]
    tunnel: w71 -> [w715]
    tunnel: w45 -> [w710]
    tunnel: w3 -> [w698]
    i -> [w716]
    stop <- w709 stop-if-true
    n157 = Greater?(x=w716, y=w715) -> (0:→"CBV Cam":bool)
    n158 = call <vilib>:"IMAQ Extract Buffer.vi"("error in (no error)"=w743, "Buffer to extract"=w716, "IMAQ Session In"=w742) -> ("error out"=w736:errorcluster, "Buffer Number"=w711:i32, "Image Out"=w713:T1, "IMAQ Session Out"=w721:refnum<k11>)  [unwired: 5 out]
    "Last CBV\nBuffer" <- w711
    "?" <- w713
    n159 = Multiply(x=w710, y=w711) -> (x*y=w712:dbl)
    n160 = Round Toward -Infinity(1:w712) -> (0:w697:dbl)
    n161 = Tick Count (ms)() -> (millisecond timer value=w735:u32)
    n162 = call <vilib>:"Calculate Frames per Second.vi"("Update Interval (ms)"=u32 2000, "Buffer Number"=w711) -> ("Processed Frames/s"=→"CBV Cam":dbl)  [unwired: 7 in, 2 out]
    n163 = Index Array(array=w698, index (row)=3, index (col)=w697) -> (element=w708:dbl)
    n164 = Index Array(array=w698, index (row)=2, index (col)=w697) -> (element=w693:dbl)
    n165 = Index Array(array=w698, index (row)=1, index (col)=w697) -> (element=w692:dbl)
    n166 = Index Array(array=w698, index (row)=0, index (col)=w697) -> (element=w691:dbl)
    n167 = Greater Or Equal?(x=w711, y=w729) -> (x >= y?=w719:bool)
    n168 = call "IMAQ ImageToArray"("error in (no error)"=w736, "Image"=w713) -> ("error out"=w741:errorcluster, "Image Pixels (I16)"=w740:i16[][])  [unwired: 2 in, 3 out]
    n169 = Subtract(x=w735, y=w730) -> (x-y=w734:u32)
    n170 = local write "stop"("stop") -> ()
    n171 = Greater?(x=w708, y=0.0) -> (0:→"Auditory":bool)
    n172 = Greater?(x=w693, y=0.0) -> (0:→"RPad":bool)
    n173 = Greater?(x=w692, y=0.0) -> (0:→"LPad":bool)
    n174 = Greater?(x=w691, y=0.0) -> (0:→"LED":bool)
    n175 = Multiply(x=w734, y=1.667e-05) -> (x*y=w733:dbl)
    n176 = Write to Binary File(file (use dialog)=w720, data=w740, error in=w741, 5:FALSE ("prepend array or string size? (T)"), 9:T11."big-endian, network order" ("byte order (0:big-endian, network order)")) -> (refnum out=w737:refnum<file>, error out=w723:errorcluster)  [unwired: 1 in, 1 out]
    n177 = Bundle("Time (min)"=w728, w733) -> (→"Time Elapsed (Min)":cluster{"Time (min)":dbl, dbl})  [unwired: 1 in]
    n178 = Compound Arithmetic op=OR(w723, w719, "stop") -> (w709:bool)
    "CBV Camera" <- w709
    "Finished" <- w709
  }
  n179 = while {
    tunnel: w426 -> [w770]
    tunnel: [w771] -> w425
    tunnel: w424 -> [w771]
    tunnel: [w770] -> w423
    tunnel: [w763] -> w286
    tunnel: [w764] -> w343
    tunnel: [w769] -> w422
    tunnel: w421 -> [w768]
    tunnel: w419 -> [w767]
    tunnel: w417 -> [w766]
    tunnel: w415 -> [w765]
    shift-right: [w754] -> _
    shift-left: _ -> [w752]
    shift-right: [w749] -> _
    shift-left: u32 0 ("New Lost") -> [w753]
    shift-right: [w750] -> w278
    shift-left: u32[] [] ("NewBuffNum") -> [w751]
    shift-right: [w756] -> w367
    shift-left: u32[] [] ("NewNumLost") -> [w755]
    tunnel: w166 -> [w761]
    tunnel: w71 -> [w757]
    i -> [w744]
    stop <- w760 stop-if-true
    n180 = call <vilib>:"IMAQdx Get Image.vi"("Buffer Number Mode (Next)"=IMAQdx_Buffer_Number_Mode."Buffer Number", "error in"=w767, "Buffer Number In"=w744, "Image In"=w766, "Session In"=w768) -> ("error out"=w777:errorcluster, "Buffer Number Out"=w754:u32, "Image Out"=w746:T1, "Session Out"=w763:T4)  [unwired: 3 in]
    "Last Whisk\nBuffer" <- w754
    "?" <- w746
    n181 = Greater?(x=w744, y=w757) -> (0:→"Whisk Cam":bool)
    n182 = call "IMAQ ImageToArray"("error in (no error)"=w777, "Image"=w746) -> ("error out"=w776:errorcluster, "Image Pixels (U8)"=w775:u8[][])  [unwired: 2 in, 3 out]
    n183 = call "TrackWhiskDroppedFrames_IOS.vi"("NumLost"=w755, "BuffNum"=w751, "Curr Buffer"=w754, "Prev Lost"=w753, "Prev Buffer"=w752) -> ("New Lost"=w749:u32, "NewNumLost"=w756:u32[], "NewBuffNum"=w750:u32[])  [unwired: 4 in]
    "Dropped" <- w749
    n184 = Add(x=w754, y=w753) -> (x+y=w762:u32)
    n185 = Greater Or Equal?(x=w762, y=w761) -> ()  [unwired: 1 out]
    n186 = Write to Binary File(file (use dialog)=w765, data=w775, error in=w776, 5:FALSE ("prepend array or string size? (T)"), 9:T11."little-endian" ("byte order (0:big-endian, network order)")) -> (refnum out=w769:refnum<file>, error out=w764:errorcluster)  [unwired: 1 in, 1 out]
    n187 = local read "stop"() -> (w748:bool)
    n188 = local read "CBV Camera"() -> (w747:bool)
    n189 = call <vilib>:"Calculate Frames per Second.vi"("Update Interval (ms)"=u32 2000, "Buffer Number"=w754) -> ("Processed Frames/s"=→"Whisk Cam Fs":dbl)  [unwired: 7 in, 2 out]
    n190 = Unbundle By Name(w764) -> ("status"=w745:bool)
    n191 = Compound Arithmetic op=OR(w745, w748, w747) -> (w760:bool)
  }
  n192 = while {
    tunnel: w442 -> [w795]
    tunnel: w436 -> [w793]
    tunnel: w434 -> [w792]
    tunnel: w432 -> [w791]
    tunnel: w429 -> [w789]
    tunnel: [w790] -> w179
    tunnel: [w781] -> w427
    tunnel: [w789] -> w428
    tunnel: w71 -> [w784]
    i -> [w785]
    stop <- w782 stop-if-true
    n193 = Tick Count (ms)() -> (millisecond timer value=w797:u32)
    n194 = Subtract(x=w797, y=w795) -> (x-y=w798:u32)
    n195 = Divide(x=w798, y=u32 1000) -> (x/y=w794:dbl)
    n196 = Greater?(x=w785, y=w784) -> (0:→"Web Cam":bool)
    n197 = call "GrabWebCam_IOS.vi"("Session In"=w792, "Image In"=w793, "Trial Time"=w794, "AVI Refnum"=w789, "error in"=w791) -> ("Session Out"=w790:T4, "WebCam Img Out"=→"?":T1, "Buffer Number Out"=w788:u32, "error out"=w781:errorcluster)  [unwired: 7 in]
    n198 = local read "CBV Camera"() -> (w783:bool)
    n199 = local read "stop"() -> (w780:bool)
    n200 = call <vilib>:"Calculate Frames per Second.vi"("Update Interval (ms)"=u32 5000, "Buffer Number"=w788) -> ("Processed Frames/s"=→"Web Cam Fs":dbl)  [unwired: 7 in, 2 out]
    n201 = Compound Arithmetic op=OR(w781, w780, w783) -> (w782:bool)
  }
  n202 = while {
    tunnel: w385 -> [w822]
    tunnel: w384 -> [w821]
    tunnel: w99 -> [w820]
    tunnel: [w819] -> w139
    tunnel: [w808] -> w138
    tunnel: [w818] -> w381
    shift-right: [w812] -> _
    shift-left: w71 -> [w803]
    tunnel: [w808] -> w229
    tunnel: w100 -> [w806]
    i -> [w804]
    stop <- w809 stop-if-true
    n203 = To Long Integer(number=w806) -> (32bit integer=w807:i32)
    n204 = call-poly <vilib>:"DAQmx Read.vi"("task/channels in"=w821, "error in"=w822) -> ("task out"=w818:refnum<k21>, "data"=w800:waveform(dbl)[], "error out"=w811:errorcluster)  [unwired: 11 in]
    n205 = Greater?(x=w803, y=w804) -> (0:→"Dev1 Analog":bool)
    n206 = TDMS Write(0:w820, 5:"Analog Data" ("group name in (Untitled)"), 9:w800, 11:w811) -> (4:w819:refnum<k34>, 15:w808:errorcluster)  [unwired: 2 in, 2 out]
    n207 = Index Array(array=w800, index=0) -> (element=w815:waveform(dbl))
    n208 = Unbundle By Name(w815) -> ("Y"=w814:dbl[])
    n209 = local read "CBV Camera"() -> (w802:bool)
    n210 = local read "stop"() -> (w801:bool)
    n211 = Array Size(array=w814) -> (size(s)=w813:i32)
    n212 = Add(x=w813, y=w803) -> (x+y=w812:i32)
    "Dev1 Samples" <- w812
    n213 = Greater Or Equal?(x=w812, y=w807) -> (x >= y?=w810:bool)
    n214 = Compound Arithmetic op=OR(w808, w810, w801, w802) -> (w809:bool)
  }
  n215 = while {
    tunnel: w97 -> [w845]
    tunnel: w98 -> [w844]
    tunnel: [w843] -> w83
    tunnel: [w832] -> w84
    tunnel: [w842] -> w94
    shift-right: [w836] -> _
    shift-left: w71 -> [w827]
    tunnel: [w832] -> w93
    tunnel: w100 -> [w830]
    tunnel: w74 -> [w824]
    i -> [w828]
    stop <- w833 stop-if-true
    n216 = To Long Integer(number=w830) -> (32bit integer=w831:i32)
    n217 = call-poly <vilib>:"DAQmx Read.vi"("task/channels in"=w844, "error in"=w845) -> ("task out"=w842:refnum<k21>, "data"=w823:waveform(dbl)[], "error out"=w835:errorcluster)  [unwired: 11 in]
    n218 = Greater?(x=w827, y=w828) -> (0:→"Dev2 Analog":bool)
    n219 = TDMS Write(0:w824, 5:"Analog Data" ("group name in (Untitled)"), 9:w823, 11:w835) -> (4:w843:refnum<k34>, 15:w832:errorcluster)  [unwired: 2 in, 2 out]
    n220 = Index Array(array=w823, index=0) -> (element=w839:waveform(dbl))
    n221 = Unbundle By Name(w839) -> ("Y"=w838:dbl[])
    n222 = local read "CBV Camera"() -> (w826:bool)
    n223 = local read "stop"() -> (w825:bool)
    n224 = Array Size(array=w838) -> (size(s)=w837:i32)
    n225 = Add(x=w837, y=w827) -> (x+y=w836:i32)
    "Dev2 Samples" <- w836
    n226 = Greater Or Equal?(x=w836, y=w831) -> (x >= y?=w834:bool)
    n227 = Compound Arithmetic op=OR(w832, w834, w825, w826) -> (w833:bool)
  }
  n228 = while {
    tunnel: [w848] -> w44
    tunnel: w2 -> [w848]
    tunnel: w1 -> [w847]
    tunnel: [w847] -> w43
    stop <- w846 stop-if-true
    n229 = local read "Finished"() -> (w846:bool)
  }
  n230 = call <vilib>:"DAQmx Stop Task.vi"("task/channels in"=w94, "error in"=w93) -> ("task out"=w96:refnum<k21>, "error out"=w95:errorcluster)  [unwired: 12 in]
  n231 = call <vilib>:"DAQmx Stop Task.vi"("task/channels in"=w381, "error in"=w229) -> ("task out"=w345:refnum<k21>, "error out"=w344:errorcluster)  [unwired: 12 in]
  n232 = call <vilib>:"IMAQ Extract Buffer.vi"("error in (no error)"=w454, "Buffer to extract"=-1, "IMAQ Session In"=w455) -> ("error out"=w476:errorcluster, "IMAQ Session Out"=w475:refnum<k11>)  [unwired: 7 out]
  n233 = Close File(refnum=w453, error in=w138) -> (path=w361:path)  [unwired: 1 out]
  n234 = Delete From Array(array=w278, length=1, index=0) -> (array with subset deleted=w241:u32[])  [unwired: 1 out]
  n235 = call-poly <vilib>:"DAQmx Write.vi"("task/channels in"=w266, "data"=FALSE, "error in"=w264) -> ("task out"=w263:refnum<k21>, "error out"=w261:errorcluster)  [unwired: 10 in, 1 out]
  n236 = Delete From Array(array=w367, length=1, index=0) -> (array with subset deleted=w242:u32[])  [unwired: 1 out]
  n237 = call <vilib>:"DAQmx Stop Task.vi"("task/channels in"=w149, "error in"=w150) -> ("task out"=w130:refnum<k21>, "error out"=w131:errorcluster)  [unwired: 12 in]
  n238 = call <vilib>:"DAQmx Stop Task.vi"("task/channels in"=w423, "error in"=w425) -> ("task out"=w128:refnum<k21>, "error out"=w129:errorcluster)  [unwired: 12 in]
  n239 = Delete From Array(array=w145, length=1, index=0) -> (array with subset deleted=w152:u32[])  [unwired: 1 out]
  n240 = Delete From Array(array=w144, length=1, index=0) -> (array with subset deleted=w151:u32[])  [unwired: 1 out]
  n241 = call <vilib>:"IMAQdx Close Camera.vi"("error in"=w343, "Session In"=w286) -> ()  [unwired: 9 in, 1 out]
  n242 = Close File(refnum=w422, error in=w343) -> (path=w359:path, error out=w358:errorcluster)
  n243 = call "IMAQ AVI2 Close"("error in (no error)"=w427, "AVI Refnum"=w428) -> ("error out"=w360:errorcluster)  [unwired: 9 in]
  n244 = call <vilib>:"IMAQdx Close Camera.vi"("error in"=w427, "Session In"=w179) -> ()  [unwired: 9 in, 1 out]
  n245 = call <vilib>:"DAQmx Clear Task.vi"("task in"=w96, "error in"=w95) -> ()  [unwired: 13 in, 1 out]
  n246 = call <vilib>:"IMAQdx Close Camera.vi"("error in"=w148, "Session In"=w147) -> ()  [unwired: 9 in, 1 out]
  n247 = Close File(refnum=w146, error in=w148) -> (path=w141:path, error out=w140:errorcluster)
  n248 = Build Array(w241, w242) -> (w244:u32[][])
  n249 = call <vilib>:"DAQmx Clear Task.vi"("task in"=w345, "error in"=w344) -> ()  [unwired: 13 in, 1 out]
  n250 = call <vilib>:"DAQmx Stop Task.vi"("task/channels in"=w263, "error in"=w261) -> ("task out"=w262:refnum<k21>, "error out"=w260:errorcluster)  [unwired: 12 in]
  n251 = call <vilib>:"DAQmx Stop Task.vi"("task/channels in"=w406, "error in"=w404) -> ("task out"=w132:refnum<k21>, "error out"=w133:errorcluster)  [unwired: 12 in]
  n252 = call <vilib>:"IMAQ Close.vi"("error in (no error)"=w476, "IMAQ Session In"=w475) -> ("error out"=w477:errorcluster)  [unwired: 9 out]
  n253 = Build Array(w151, w152) -> (w154:u32[][])
  n254 = call <vilib>:"DAQmx Clear Task.vi"("task in"=w128, "error in"=w129) -> ()  [unwired: 13 in, 1 out]
  n255 = call <vilib>:"DAQmx Clear Task.vi"("task in"=w130, "error in"=w131) -> ()  [unwired: 13 in, 1 out]
  n256 = Array To Spreadsheet String(delimiter (Tab)=",", array=w242, 3:"%d" ("format string")) -> (spreadsheet string=w279:string)
  n257 = Transpose 2D Array(2D array=w244) -> (transposed array=w243:u32[][])
  n258 = Array To Spreadsheet String(delimiter (Tab)=",", array=w241, 3:"%d" ("format string")) -> (spreadsheet string=w280:string)
  n259 = Move(source path=w141, error in=w140, 10:"Target Path") -> (error out=w142:errorcluster)  [unwired: 2 in, 2 out]
  n260 = Move(source path=w359, error in=w358, 10:"Target Path") -> (error out=w356:errorcluster)  [unwired: 2 in, 2 out]
  n261 = call <vilib>:"DAQmx Stop Task.vi"("task/channels in"=w44, "error in"=w43) -> ("task out"=w55:refnum<k21>, "error out"=w54:errorcluster)  [unwired: 12 in]
  n262 = Array To Spreadsheet String(delimiter (Tab)=",", array=w152, 3:"%d" ("format string")) -> (spreadsheet string=w155:string)
  n263 = Transpose 2D Array(2D array=w154) -> (transposed array=w153:u32[][])
  n264 = Array To Spreadsheet String(delimiter (Tab)=",", array=w151, 3:"%d" ("format string")) -> (spreadsheet string=w156:string)
  n265 = Move(source path=w41, error in=w360, 10:"Target Path") -> (error out=w355:errorcluster)  [unwired: 2 in, 2 out]
  n266 = call <vilib>:"DAQmx Clear Task.vi"("task in"=w132, "error in"=w133) -> ()  [unwired: 13 in, 1 out]
  n267 = TDMS Close(8:w84, 11:w83) -> (0:w92:errorcluster, 3:w72:path)
  n268 = call <vilib>:"DAQmx Clear Task.vi"("task in"=w262, "error in"=w260) -> ()  [unwired: 13 in, 1 out]
  n269 = for {
    N: w231 -> [_]
    tunnel: w471 -> [w852] mode=indexing
    shift-right: [w850] -> w363
    shift-left: w477 -> [w851]
    n270 = call "IMAQ Dispose"("All Images? (No)"=FALSE, "Image"=w852, "error in (no error)"=w851) -> ("error out"=w850:errorcluster)  [unwired: 3 out]
  }
  n271 = call <vilib>:"Trim Whitespace.vi"("string"=w280) -> ("trimmed string"=w124:string)  [unwired: 1 in]
  n272 = call <vilib>:"Trim Whitespace.vi"("string"=w279) -> ("trimmed string"=w123:string)  [unwired: 1 in]
  n273 = Number To Decimal String(number=w243) -> ()  [unwired: 1 in, 1 out]
  n274 = call <vilib>:"Trim Whitespace.vi"("string"=w156) -> ("trimmed string"=w125:string)  [unwired: 1 in]
  n275 = call <vilib>:"Trim Whitespace.vi"("string"=w155) -> ("trimmed string"=w126:string)  [unwired: 1 in]
  n276 = Number To Decimal String(number=w153) -> ()  [unwired: 1 in, 1 out]
  n277 = call <vilib>:"Simple Error Handler.vi"("error in (no error)"=w142) -> ()  [unwired: 1 in, 8 out]
  n278 = call <vilib>:"Simple Error Handler.vi"("error in (no error)"=w356) -> ()  [unwired: 1 in, 8 out]
  n279 = call <vilib>:"DAQmx Clear Task.vi"("task in"=w55, "error in"=w54) -> ()  [unwired: 13 in, 1 out]
  n280 = Path To String(path=w72) -> (string=w90:string)
  n281 = call <vilib>:"Simple Error Handler.vi"("error in (no error)"=w355) -> ()  [unwired: 1 in, 8 out]
  n282 = TDMS Defragment(4:w92, 7:w72) -> (0:w86:errorcluster)
  n283 = Build Array(w125, w126, w124, w123) -> (w122:string[])
  n284 = Concatenate Strings(w90, "_index" ("string")) -> (w88:string)
  n285 = Move(source path=w361, error in=w363, 10:"Target Path") -> (error out=w362:errorcluster)  [unwired: 2 in, 2 out]
  n286 = String To Path(string=w88) -> (path=w87:path)
  n287 = call <vilib>:"Simple Error Handler.vi"("error in (no error)"=w362) -> ()  [unwired: 1 in, 8 out]
  n288 = Move(source path=w72, error in=w86, 10:"Target Path") -> (error out=w91:errorcluster)  [unwired: 2 in, 2 out]
  n289 = Move(source path=w87, error in=w86, 10:"Target Path") -> (error out=w85:errorcluster)  [unwired: 2 in, 2 out]
  n290 = TDMS Set Properties(5:w122, 7:string[] ["PupilCam_DroppedFrameIndex", "PupilCam_NumberDropped", "WhiskCam_DroppedFrameIndex", "WhiskCam_NumberDropped"] ("channel name(s) in (Untitled)"), 8:w138, 11:w139) -> (0:w287:errorcluster, 3:w285:refnum<k34>)  [unwired: 2 in, 2 out]
  n291 = call <vilib>:"Simple Error Handler.vi"("error in (no error)"=w91) -> ()  [unwired: 1 in, 8 out]
  n292 = call <vilib>:"Simple Error Handler.vi"("error in (no error)"=w85) -> ()  [unwired: 1 in, 8 out]
  n293 = TDMS Close(8:w287, 11:w285) -> (0:w364:errorcluster, 3:w352:path)
  n294 = Path To String(path=w352) -> (string=w354:string)
  n295 = TDMS Defragment(4:w364, 7:w352) -> (0:w349:errorcluster)
  n296 = Concatenate Strings(w354, "_index" ("string")) -> (w351:string)
  n297 = String To Path(string=w351) -> (path=w350:path)
  n298 = Move(source path=w352, error in=w349, 10:"Target Path") -> (error out=w357:errorcluster)  [unwired: 2 in, 2 out]
  n299 = Move(source path=w350, error in=w349, 10:"Target Path") -> (error out=w143:errorcluster)  [unwired: 2 in, 2 out]
  n300 = call <vilib>:"Simple Error Handler.vi"("error in (no error)"=w357) -> ()  [unwired: 1 in, 8 out]
  n301 = call <vilib>:"Simple Error Handler.vi"("error in (no error)"=w143) -> ()  [unwired: 1 in, 8 out]
